vi "SubsystemControl.vi"(5 "Max Timeout(s)":dbl, 7 "Timeout":i32, 8 "error in (no error)":errorcluster, 10 "SubsystemData.lvclass":refnum<class "SubsystemData.lvclass">, 11 "Subsystem in":refnum<class "Subsystem.lvclass">) -> (0 "error out":errorcluster, 3 "Subsystem out":refnum<class "Subsystem.lvclass">)   [LabVIEW 2017, in "Subsystem.lvclass"]
uses:
  Subsystem.lvclass
  SubsystemData/SubsystemData.lvclass
  GetQueueRef.ctl
  Subsystem.lvclass/Subsystem.ctl
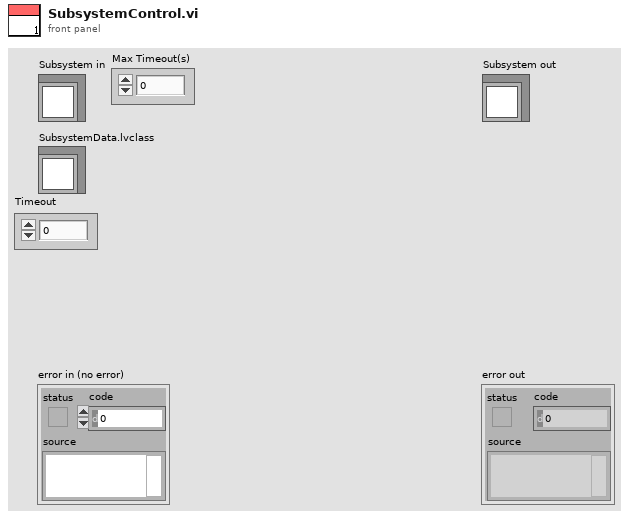
[diagram p1: front panel]
types:
  T1 = typedef "Subsystem.lvclass/GetQueueRef.ctl" = enum16{"Both", "Command", "Output"}
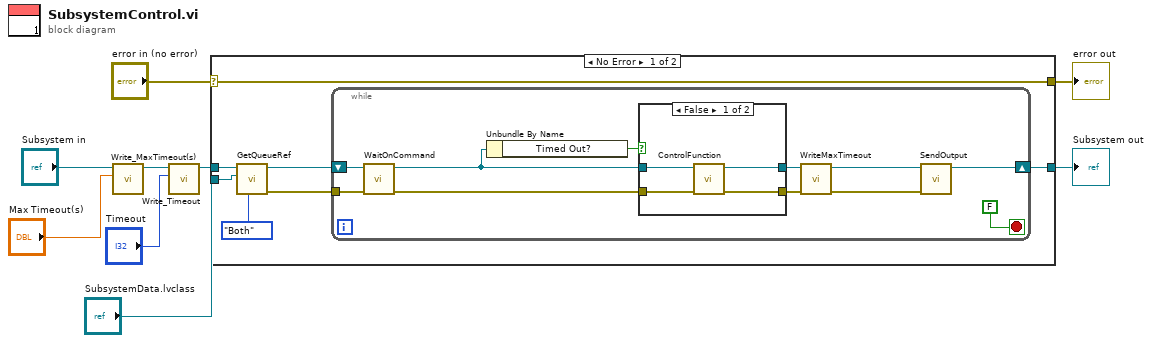
[diagram p0: block diagram]
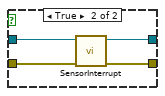
[diagram p2: hidden frame]
diagram:
  n1 = call-dynamic "Write_MaxTimeout(s).vi"("Max Timeout(s)"="Max Timeout(s)", "Subsystem in"="Subsystem in") -> ("Subsystem out"=w5:refnum<class "Subsystem.lvclass">)  [unwired: 8 in, 1 out]
  n2 = call-dynamic "Write_Timeout.vi"("Timeout"="Timeout", "Subsystem in"=w5) -> ("Subsystem out"=w3:refnum<class "Subsystem.lvclass">)  [unwired: 8 in, 1 out]
  n3 = case shown="No Error" "error in (no error)" {
    selector: "error in (no error)" -> [w16 w37]
    tunnel: [w16 w37] -> w8
    tunnel: [w13 w36] -> w7
    tunnel: w3 -> [w15 w36]
    tunnel: "SubsystemData.lvclass" -> [w12 _]
    frame No Error {
      n4 = call-dynamic "GetQueueRef.vi"("GetQueueRef"=GetQueueRef."Both", "SubsystemData.lvclass"=w12, "Subsystem in"=w15) -> ("error out"=w11:errorcluster, "Subsystem out"=w14:refnum<class "Subsystem.lvclass">)  [unwired: 7 in]
      n5 = while {
        shift-right: [w17] -> w13
        shift-left: w14 -> [w26]
        tunnel: w11 -> [w25]
        stop <- FALSE stop-if-true
        n6 = call-dynamic "WaitOnCommand.vi"("error in (no error)"=w25, "Subsystem in"=w26) -> ("error out"=w24:errorcluster, "Subsystem out"=w23:refnum<class "Subsystem.lvclass">)  [unwired: 8 in]
        n7 = Unbundle By Name(w23) -> ("Timed Out?"=w22:bool)
        n8 = case shown="False" w22 {
          tunnel: [w31 w32] -> w21
          tunnel: w24 -> [w30 w34]
          tunnel: w23 -> [w29 w35]
          tunnel: [w28 w33] -> w20
          frame False {
            n9 = call-dynamic "ControlFunction.vi"("error in (no error)"=w30, "Subsystem in"=w29) -> ("error out"=w28:errorcluster, "Subsystem out"=w31:refnum<class "Subsystem.lvclass">)  [unwired: 8 in]
          }
          frame True {
            n10 = call-dynamic "SensorInterrupt.vi"("error in (no error)"=w34, "Subsystem in"=w35) -> ("error out"=w33:errorcluster, "Subsystem out"=w32:refnum<class "Subsystem.lvclass">)  [unwired: 8 in]
          }
        }
        n11 = call-dynamic "WriteMaxTimeout.vi"("error in (no error)"=w20, "Subsystem in"=w21) -> ("error out"=w18:errorcluster, "Subsystem out"=w19:refnum<class "Subsystem.lvclass">)  [unwired: 8 in]
        n12 = call-dynamic "SendOutput.vi"("error in (no error)"=w18, "Subsystem in"=w19) -> ("Subsystem out"=w17:refnum<class "Subsystem.lvclass">)  [unwired: 8 in, 1 out]
      }
    }
    frame Error {
    }
  }
  "error out" <- w8
  "Subsystem out" <- w7
